vi "AutoRocketHatch.vi"(6 "DestinationName":string, 8 "DestinationAngle":dbl, 9 "DestinationPort":dbl[](array[numeric]), 10 "FeederStation":dbl[](array[numeric]), 11 "Coordinates":dbl[](array[numeric])) -> ()   [LabVIEW 2018]
uses:
  Globals.vi
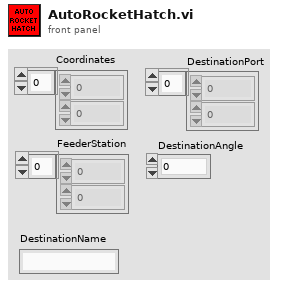
[diagram p1: front panel]
types:
  T1 = enum16{"DriveToHatch", "VisionAlign", "PlaceHatch", "DriveToFeeder"}
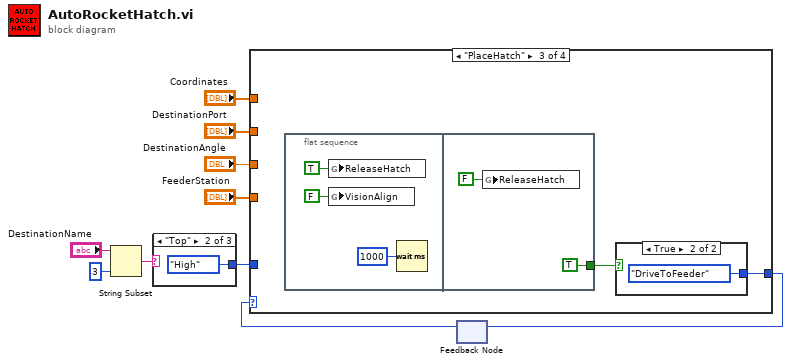
[diagram p0: block diagram]
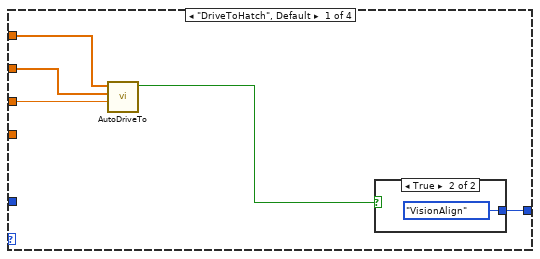
[diagram p2: hidden frame]
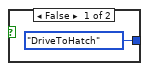
[diagram p3: hidden frame]
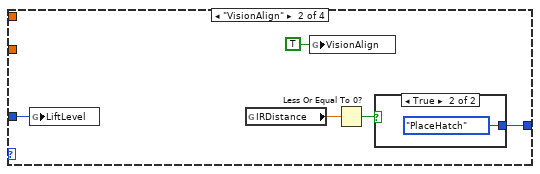
[diagram p4: hidden frame]
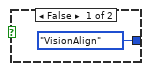
[diagram p5: hidden frame]
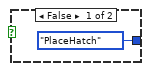
[diagram p6: hidden frame]
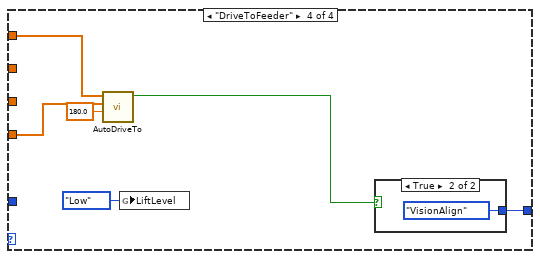
[diagram p7: hidden frame]
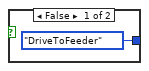
[diagram p8: hidden frame]
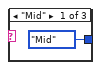
[diagram p9: hidden frame]
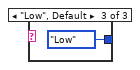
[diagram p10: hidden frame]
diagram:
  n1 = String Subset(string="DestinationName", length (rest)=3 ("length (rest)")) -> (substring=w8:string)  [unwired: 1 in]
  n2 = case shown="\"Top\"" w8 {
    tunnel: [enum16{"Low", "Mid", "High"}."Mid" ("LiftLevel") enum16{"Low", "Mid", "High"}."High" ("LiftLevel") enum16{"Low", "Mid", "High"}."Low" ("LiftLevel")] -> w4
    frame "Mid" {
    }
    frame "Top" {
    }
    frame "Low", Default {
    }
  }
  n3 = feedback #1() -> (w7:T1)  [unwired: 1 in]
  n4 = case shown="\"PlaceHatch\"" w7 {
    tunnel: "Coordinates" -> [w18 _ _ w42]
    tunnel: [w16 w22 w28 w39] -> w6
    tunnel: w4 -> [_ w21 _ _]
    tunnel: "DestinationPort" -> [w15 _ _ _]
    tunnel: "DestinationAngle" -> [w14 _ _ _]
    tunnel: "FeederStation" -> [_ _ _ w38]
    frame "DriveToHatch", Default {
      n5 = call "AutoDriveTo.vi"("EndAngle"=w14, "EndCoordinates"=w15, "Coordinates"=w18) -> ("ThereYet?"=w17:bool)  [unwired: 8 in]
      n6 = case shown="True" w17 {
        tunnel: [T1."DriveToHatch" T1."VisionAlign"] -> w16
        frame False {
        }
        frame True {
        }
      }
    }
    frame "VisionAlign" {
      n7 = global write "Globals.vi" "LiftLevel"(w21) -> ()
      n8 = global read "Globals.vi" "IRDistance"() -> (w24:dbl)
      n9 = global write "Globals.vi" "VisionAlign"(TRUE ("VisionAlign")) -> ()
      n10 = Less Or Equal To 0?(x=w24) -> (x <= 0?=w23:bool)
      n11 = case shown="True" w23 {
        tunnel: [T1."VisionAlign" T1."PlaceHatch"] -> w22
        frame False {
        }
        frame True {
        }
      }
    }
    frame "PlaceHatch" {
      n12 = flat-sequence {
        tunnel: [TRUE ("VisionAlign")] -> w29
        frame #0 {
          n13 = global write "Globals.vi" "ReleaseHatch"(TRUE ("ReleaseHatch")) -> ()
          n14 = global write "Globals.vi" "VisionAlign"(FALSE ("VisionAlign")) -> ()
          n15 = Wait (ms)(milliseconds to wait=u32 1000) -> ()  [unwired: 1 out]
        }
        frame #1 {
          n16 = global write "Globals.vi" "ReleaseHatch"(FALSE ("ReleaseHatch")) -> ()
        }
      }
      n17 = case shown="True" w29 {
        tunnel: [T1."PlaceHatch" T1."DriveToFeeder"] -> w28
        frame False {
        }
        frame True {
        }
      }
    }
    frame "DriveToFeeder" {
      n18 = call "AutoDriveTo.vi"("EndAngle"=180.0, "EndCoordinates"=w38, "Coordinates"=w42) -> ("ThereYet?"=w40:bool)  [unwired: 8 in]
      n19 = global write "Globals.vi" "LiftLevel"(enum16{"Low", "Mid", "High"}."Low" ("LiftLevel")) -> ()
      n20 = case shown="True" w40 {
        tunnel: [T1."DriveToFeeder" T1."VisionAlign"] -> w39
        frame False {
        }
        frame True {
        }
      }
    }
  }
  n21 = feedback-in #1(w6) -> ()
